vi "trapezoid.vi"() -> ()   [LabVIEW 2021]
uses:
  <vilib>/Instr/_visa.llb/VISA Configure Serial Port (Instr).vi
panel:
  in  "stop":bool
  in  "VISA resource name":refnum<visa-resource-name>="COM7"
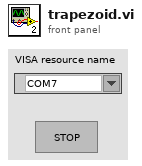
[diagram p1: front panel]
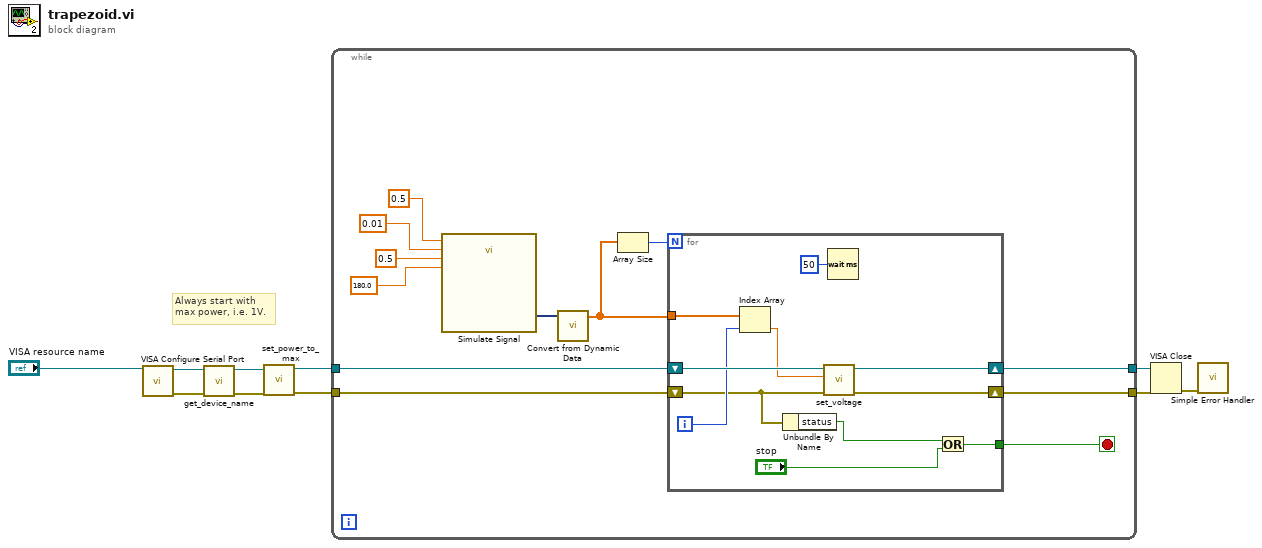
[diagram p0: block diagram]
diagram:
  # "Always start with\nmax power, i.e. 1V."
  n1 = call-poly "VISA Configure Serial Port"("VISA resource name"="VISA resource name") -> ("VISA resource name out"=w3:refnum<visa-resource-name>, "error out"=w4:errorcluster)  [unwired: 9 in, 4 out]
  n2 = call "get_device_name.vi"("error in"=w4, "VISA resource name in"=w3) -> ("error out"=w5:errorcluster, "VISA resource name out"=w6:refnum<visa-resource-name>)  [unwired: 7 in, 1 out]
  n3 = call "set_power_to_max.vi"("error in"=w5, "VISA resource name"=w6) -> ("error out"=w1:errorcluster, "VISA resource name out"=w2:refnum<visa-resource-name>)  [unwired: 8 in]
  n4 = while {
    tunnel: [w21] -> w8
    tunnel: [w22] -> w7
    tunnel: w2 -> [w20]
    tunnel: w1 -> [w19]
    stop <- w18 stop-if-true
    n5 = call "Simulate Signal"("Offset"=0.5, "Frequency"=0.01, "Amplitude"=0.5, "Phase"=180.0) -> ("Sawtooth"=w17:dynamicdata)  [unwired: 10 in, 1 out]
    n6 = call "Convert from Dynamic Data"("Dynamic Data Type"=w17) -> ("Array"=w16:dbl[])  [unwired: 3 in]
    n7 = Array Size(array=w16) -> (size(s)=w15:i32)
    n8 = for {
      N: w15 -> [_]
      shift-right: [w33] -> w22
      shift-left: w20 -> [w31]
      shift-right: [w32] -> w21
      shift-left: w19 -> [w27]
      tunnel: [w24] -> w18
      tunnel: w16 -> [w23]
      i -> [w28]
      n9 = Index Array(array=w23, index=w28) -> (element=w29:dbl)
      n10 = Unbundle By Name(w27) -> ("status"=w25:bool)
      n11 = call "set_voltage.vi"("error in"=w27, "voltage"=w29, "VISA resource name"=w31) -> ("error out"=w32:errorcluster, "VISA resource name out"=w33:refnum<visa-resource-name>)  [unwired: 6 in, 1 out]
      n12 = Wait (ms)(milliseconds to wait=u32 50) -> ()  [unwired: 1 out]
      n13 = Or(x=w25, y="stop") -> (x .or. y?=w24:bool)
    }
  }
  n14 = VISA Close(VISA resource name=w7, error in (no error)=w8) -> (error out=w9:errorcluster)
  n15 = call <vilib>:"Simple Error Handler.vi"("error in (no error)"=w9) -> ()  [unwired: 1 in, 8 out]
